vi "3_0_Linear convolution.vi"(0 "sequence x[n]":dbl[](array[numeric]), 1 "sequence h[n]":dbl[](array[numeric])) -> (2 "sequence y[n] = x[n] * h[n]":dbl[](array[numeric]), 3 "Sequence x[n]":dbl[](graph), 4 "Sequence h[n]":dbl[](graph), 5 "Sequence y[n] = x[n] * h[n]":dbl[](graph))   [LabVIEW 2009]
panel:
  # "LINEAR CONVOLUTION"
  # "Program Developed by Indranil Sinharoy"
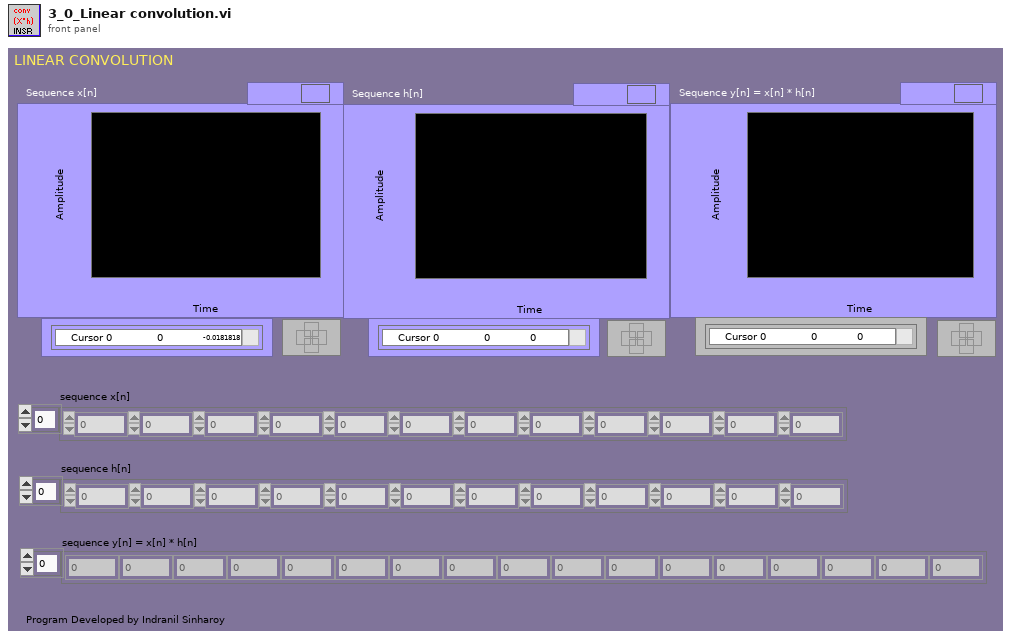
[diagram p1: front panel]
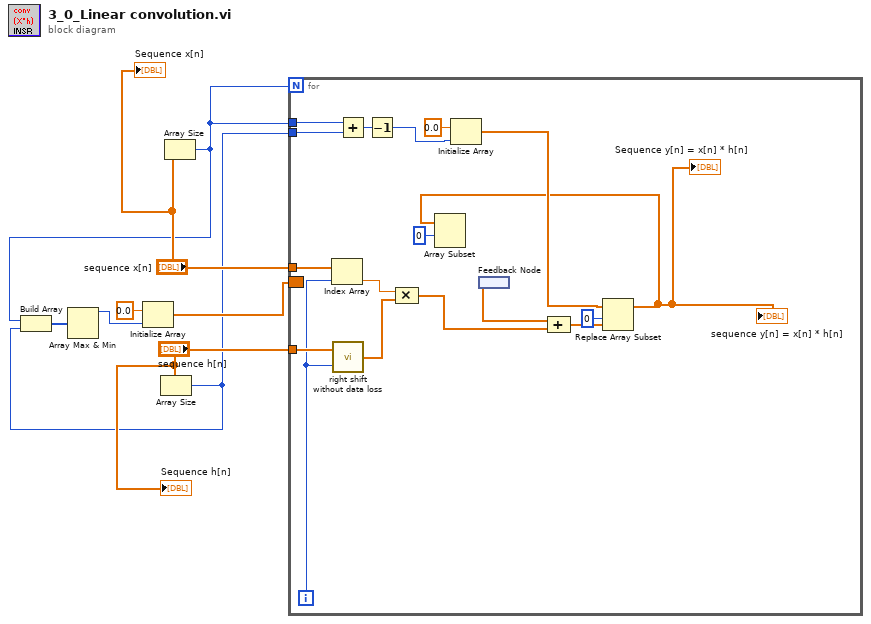
[diagram p0: block diagram]
diagram:
  n1 = Array Size(array="sequence h[n]") -> (size(s)=w3:i32)
  n2 = Array Size(array="sequence x[n]") -> (size(s)=w4:i32)
  n3 = Build Array(w4, w3) -> (w2:i32[])
  n4 = Array Max & Min(array=w2) -> (max value=w1:i32)  [unwired: 3 out]
  n5 = Initialize Array "Initialize Array"(0.0 ("element"), w1) -> (w5:dbl[])
  n6 = for {
    N: w4 -> [_]
    tunnel: "sequence h[n]" -> [w26]
    tunnel: "sequence x[n]" -> [w25]
    tunnel: w4 -> [w12]
    tunnel: w3 -> [w11]
    border: w5 -> [_]
    i -> [w22]
    n7 = Index Array "Index Array"(array=w25, index=w22) -> (element=w21:dbl)
    n8 = call "right shift without data loss.vi"("shift index"=w22, "x[n]"=w26) -> ("Right shifted x[n]"=w23:dbl[])
    n9 = Add(x=w12, y=w11) -> (x+y=w15:i32)
    n10 = Decrement(x=w15) -> (x-1=w13:i32)
    n11 = Compound Arithmetic op=MULTIPLY(w21, w23) -> (w24:dbl[])
    n12 = Initialize Array "Initialize Array"(0.0 ("element"), w13) -> (w10:dbl[])
    n13 = feedback #1() -> (w18:dbl[])
    n14 = Compound Arithmetic op=ADD(w18, w24) -> (w20:dbl[])
    n15 = Replace Array Subset "Replace Array Subset"(array=w10, new element=w20, index=0) -> (w9:dbl[])
    "sequence y[n] = x[n] * h[n]" <- w9
    "Sequence y[n] = x[n] * h[n]" <- w9
    n16 = Array Subset "Array Subset"(array=w9, index=0) -> (w19:dbl[])  [unwired: 1 in]
  }
  "Sequence x[n]" <- "sequence x[n]"
  "Sequence h[n]" <- "sequence h[n]"
